vi "Write Coded Binary Data.vi"(7 "AC Data":refnum<class "Data.lvclass">, 8 "error in":errorcluster, 9 "cell":i32=-1, 10 "binRefIn":refnum<file>, 11 "cPAS Cell in":refnum<class "cPAS Cell Data.lvclass">) -> (0 "error out":errorcluster, 3 "cPAS Cell out":refnum<class "cPAS Cell Data.lvclass">)   [LabVIEW 2014, in "cPAS Cell Data.lvclass"]
uses:
  cPAS Cell Data.lvclass
  Reusable/Data/Data.lvclass
  Read lRMS_hw.vi
  Read T2_cell.vi
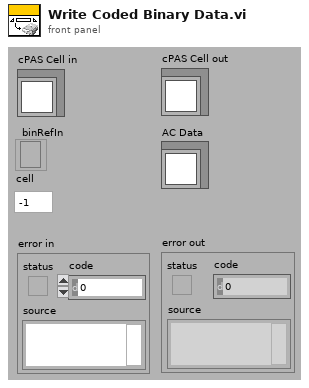
[diagram p1: front panel]
types:
  T1 = enum16{"big-endian, network order", "native, host order", "little-endian"}
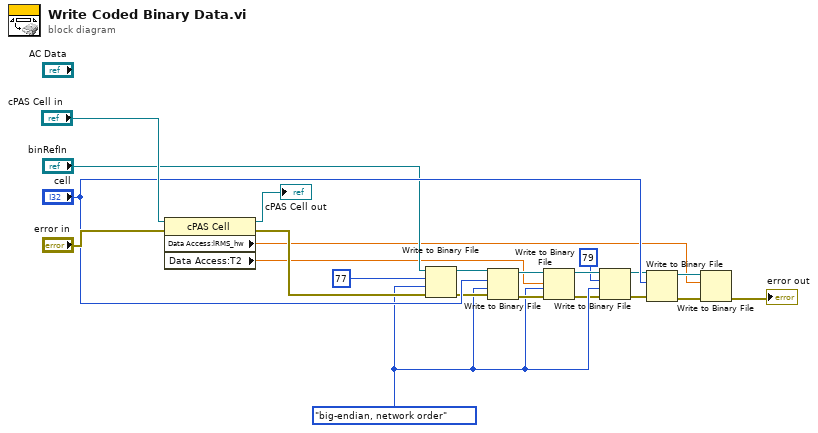
[diagram p0: block diagram]
diagram:
  w6 = T1."big-endian, network order" ("byte order (0:big-endian, network order)")
  n1 = property class="cPAS Cell"(reference="cPAS Cell in", error in="error in") -> (reference out=→"cPAS Cell out":refnum<class "cPAS Cell Data.lvclass">, error out=w17:errorcluster, "Data Access:lRMS_hw"=w2:sgl, "Data Access:T2"=w3:sgl)
  n2 = Write to Binary File(file (use dialog)="binRefIn", data=u8 77, error in=w17, 9:w6) -> (refnum out=w15:refnum<file>, error out=w14:errorcluster)  [unwired: 2 in, 1 out]
  n3 = Write to Binary File(file (use dialog)=w15, data="cell", error in=w14, 9:w6) -> (refnum out=w13:refnum<file>, error out=w12:errorcluster)  [unwired: 2 in, 1 out]
  n4 = Write to Binary File(file (use dialog)=w13, data=w3, error in=w12, 9:w6) -> (refnum out=w7:refnum<file>, error out=w5:errorcluster)  [unwired: 2 in, 1 out]
  n5 = Write to Binary File(file (use dialog)=w7, data=u8 79, error in=w5, 9:w6) -> (refnum out=w8:refnum<file>, error out=w9:errorcluster)  [unwired: 2 in, 1 out]
  n6 = Write to Binary File(file (use dialog)=w8, data="cell", error in=w9) -> (refnum out=w10:refnum<file>, error out=w11:errorcluster)  [unwired: 3 in, 1 out]
  n7 = Write to Binary File(file (use dialog)=w10, data=w2, error in=w11) -> (error out=→"error out":errorcluster)  [unwired: 3 in, 2 out]
